vi "Untitled 1.vi"() -> ()   [LabVIEW 2011]
panel:
  out "Temperatura Medie":dbl(slide) scale=0.0..100.0
  out "Grafic temperaturi":T1(graph)
  out "Comanda Incalzitor":bool
  in  "stop":bool
  out "Temperatura curenta":dbl
  out "Valoare Convertita":dbl
  in  "Limita Superioara":dbl
  in  "Limita Inferioara":dbl
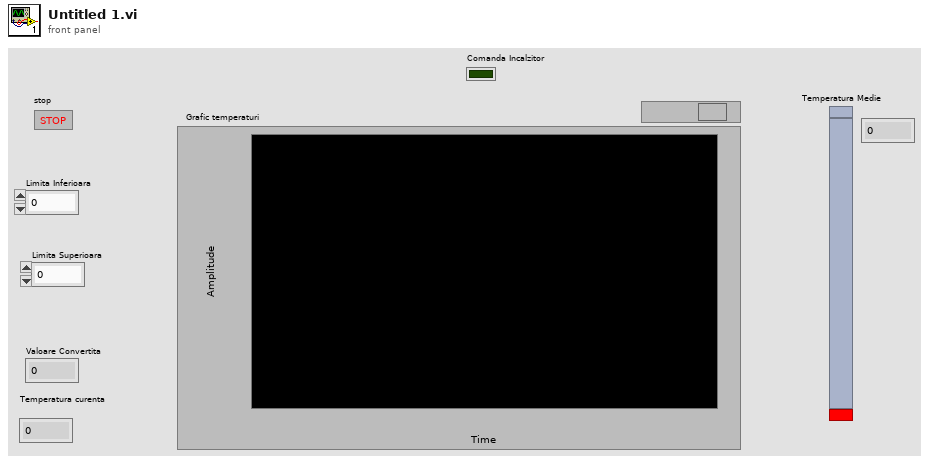
[diagram p1: front panel]
types:
  T1 = cluster{"Limita Superioara ":dbl, dbl, "Limita Inferioara":dbl, dbl}
  T2 = cluster{"Limita Superioara ":dbl, dbl, void, dbl}
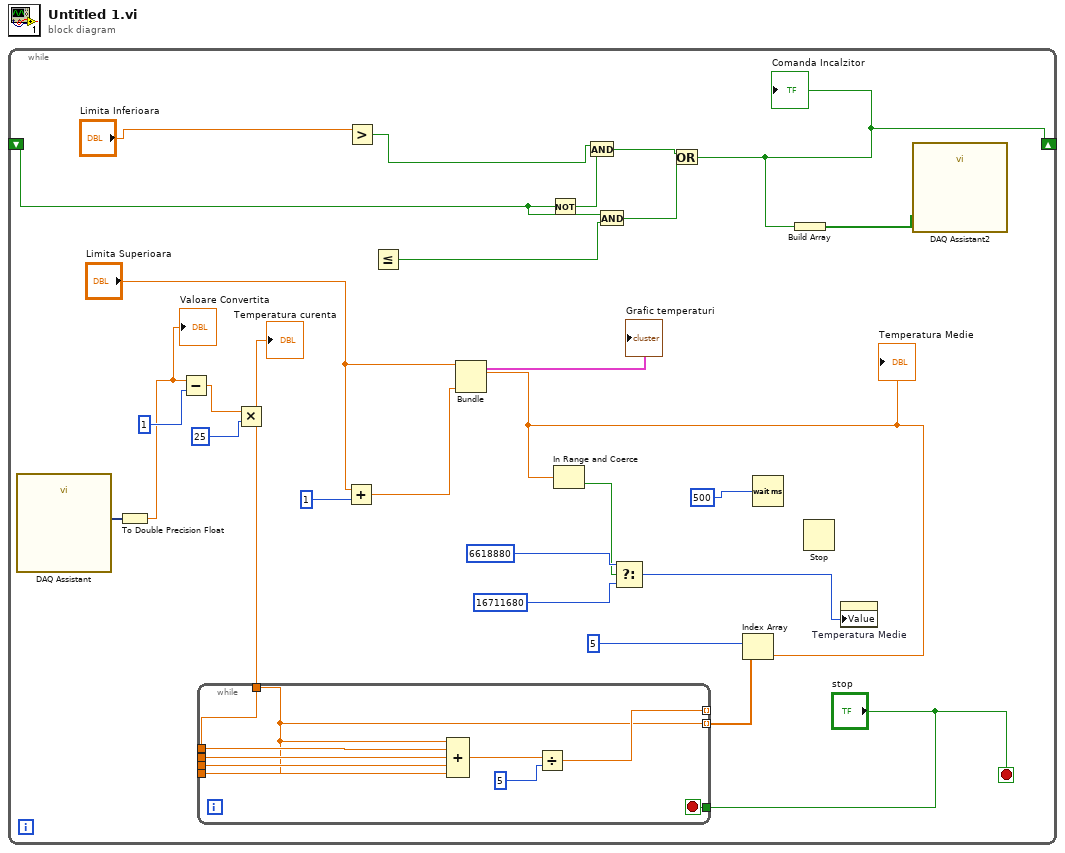
[diagram p0: block diagram]
diagram:
  n1 = while {
    shift-right: [w8] -> _
    shift-left: _ -> [w6]
    stop <- "stop" stop-if-true
    n2 = call "DAQ Assistant"() -> ("data"=w25:dynamicdata)  [unwired: 17 in, 2 out]
    n3 = To Double Precision Float(number=w25) -> (double precision float=w3:dbl)
    "Valoare Convertita" <- w3
    n4 = Subtract(x=w3, y=1) -> (x-y=w22:dbl)
    n5 = Multiply(x=w22, y=25) -> (x*y=w9:dbl)
    "Temperatura curenta" <- w9
    n6 = while {
      tunnel: [w35] -> _ mode=indexing
      tunnel: [w31] -> w11 mode=indexing
      tunnel: w9 -> [w34]
      tunnel: w9 -> [w33]
      tunnel: w9 -> [w32]
      tunnel: [w31] -> _
      tunnel: w9 -> [w31]
      tunnel: "stop" -> [w30]
      stop <- w30 stop-if-true
      n7 = Compound Arithmetic op=unknown(w31, w34, w32, w33, w31) -> (w36:dbl)
      n8 = Divide(x=w36, y=5) -> (x/y=w35:dbl)
    }
    n9 = Add(x="Limita Superioara", y=1) -> (x+y=w16:dbl)
    n10 = Greater?(x="Limita Inferioara") -> (0:w7:bool)  [unwired: 1 in]
    n11 = Less Or Equal?() -> (x <= y?=w21:bool)  [unwired: 2 in]
    n12 = Not(x=w6) -> (.not. x?=w5:bool)
    n13 = And(x=w7, y=w5) -> (x .and. y?=w20:bool)
    n14 = And(x=w6, y=w21) -> (x .and. y?=w19:bool)
    n15 = Or(x=w20, y=w19) -> (x .or. y?=w8:bool)
    "Comanda Incalzitor" <- w8
    n16 = Index Array(array=w11, index=5) -> (element=w2:dbl)
    "Temperatura Medie" <- w2
    n17 = Bundle("Limita Superioara"="Limita Superioara", w2, w16) -> (→"Grafic temperaturi":T2)  [unwired: 2 in]
    n18 = In Range and Coerce(x=w2) -> (In Range?=w14:bool)  [unwired: 2 in, 1 out]
    n19 = Select(t=6618880, s=w14, f=16711680) -> (s? t:f=w13:i32)
    n20 = Wait (ms)(milliseconds to wait=500) -> ()  [unwired: 1 out]
    n21 = Build Array(w8) -> (w18:bool[])
    n22 = Stop() -> ()  [unwired: 1 in]
    n23 = property on="Temperatura Medie" class="Slide (strict)"("Value"=w13) -> ()  [unwired: 2 in, 2 out]
    n24 = call "DAQ Assistant2"("data"=w18) -> ()  [unwired: 17 in, 2 out]
  }
